vi "Generate Waveform.vi"(0 "number of samples":u32=300000 caption="Number of Samples", 5 "sample rate [S/s]":dbl=10000000.0 caption="Sample Rate [S/s]" format="%#.3pS/s", 7 "tone frequency":dbl=130000.0 caption="Tone Frequency [Hz]" format="%#.3pHz", 9 "Amplitude":dbl=0.5 format="%0.2p") -> (4 "I":i16[](array[numeric]), 6 "Q":i16[](array[numeric]), 8 "Waveform":waveform(dbl)[](graph))   [LabVIEW 2017]
doc: "Create a waveform to send to a device for generation.\n\n<B>Input Parameters</B>\n\n<B>tone frequency</B> is the frequency of the tone (in Hertz) to generate.\n\n<B>number of samples</B> is the number of samples in the generated waveform.\n\n<B>sample rate [S/s]</B> is the sample rate (in samples per second) that will be used during generation.\n\n<B>Amplitude</B> is used to set the amplitude of the tone.\n\n<B>Output Parameters</B>\n\n<B>Waveform</B> is the generated waveform.\n\n<B>I</B> is the real (I) portion of the generated waveform.\n\n<B>Q</B> is the imaginary (Q) portion of the generated waveform."
uses:
  <vilib>/measure/NI_MABase.lvlib
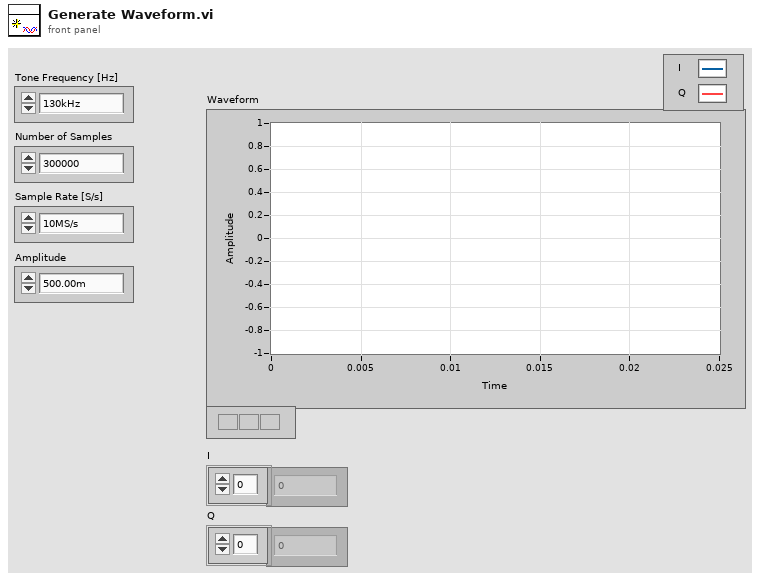
[diagram p1: front panel]
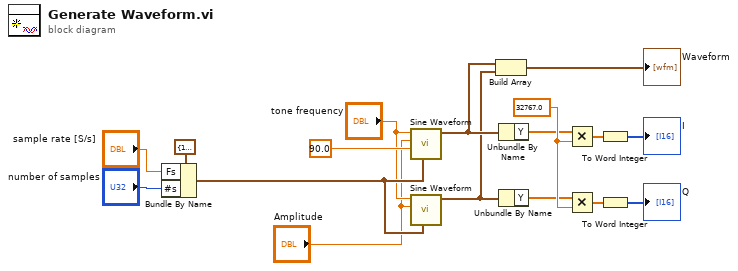
[diagram p0: block diagram]
diagram:
  w13 = 32767.0
  n1 = Bundle By Name(cluster=cluster{"Fs":dbl, "#s":dbl} {"Fs"=1000.0, "#s"=1000.0} ("sampling info"), "Fs"="sample rate [S/s]", "#s"="number of samples") -> (w9:cluster{"Fs":dbl, "#s":dbl})
  n2 = call <vilib>:"Sine Waveform.vi"("sampling info"=w9, "phase"=90.0, "amplitude"="Amplitude", "frequency"="tone frequency") -> ("signal out"=w7:waveform(dbl))  [unwired: 6 in, 1 out]
  n3 = call <vilib>:"Sine Waveform.vi"("sampling info"=w9, "amplitude"="Amplitude", "frequency"="tone frequency") -> ("signal out"=w6:waveform(dbl))  [unwired: 7 in, 1 out]
  n4 = Build Array(w7, w6) -> (→"Waveform":waveform(dbl)[])
  n5 = Unbundle By Name(w7) -> ("Y"=w11:dbl[])
  n6 = Unbundle By Name(w6) -> ("Y"=w12:dbl[])
  n7 = Multiply(x=w11, y=w13) -> (x*y=w14:dbl[])
  n8 = Multiply(x=w12, y=w13) -> (x*y=w15:dbl[])
  n9 = To Word Integer(number=w14) -> (16bit integer=→"I":i16[])
  n10 = To Word Integer(number=w15) -> (16bit integer=→"Q":i16[])
